vi "Execute.vi"(8 "error in (no error)":errorcluster, 11 "Node in":refnum<class "Set Double Float.lvclass">) -> (0 "error out":errorcluster, 1 "Status":T1, 3 "Node out":refnum<class "Set Double Float.lvclass">)   [LabVIEW 2021, in "BT.lvlib" / "Set Double Float.lvclass"]
uses:
  Set Double Float.lvclass
  C:/Users/Tim/Documents/GitHub/LV_Behaviour_Tree/BT Abstract Type/abs_Type Leaf/abs_Type Leaf.lvclass
  abs_Node/Status.ctl
  <vilib>/TSA/Abstract Data Classes/Abs_Types/Double Float/Abs_Double Float.lvclass
  C:/Program Files (x86)/National Instruments/LabVIEW 2021/vi.lib/TSA/Abstract Data Classes/Abs_Types/Type/Abs_Type.lvclass
  abs_Type Leaf/abs_Type Leaf.lvclass/abs_Type Leaf.ctl
  Set Double Float.lvclass/Set Double Float.ctl
  abs_Type Leaf/Properties/Read Value Class.vi
  Properties/Read Value.vi
  abs_Type Leaf/Properties/Write Value Class.vi
  <vilib>/TSA/Abstract Data Classes/Abs_Types/Type/Abs_Type.lvclass
  abs_Type Leaf/abs_Type Leaf.lvclass
  abs_Node/bt_Node.lvclass
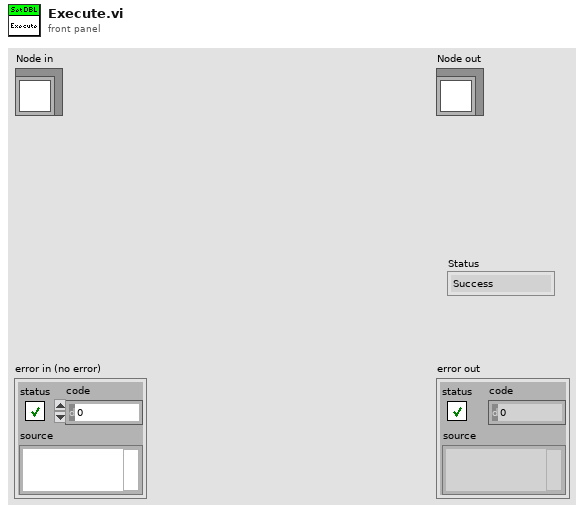
[diagram p1: front panel]
types:
  T1 = typedef "BT.lvlib/bt_Node.lvclass/Status.ctl" = enum16{"Success", "Failure", "Running"}
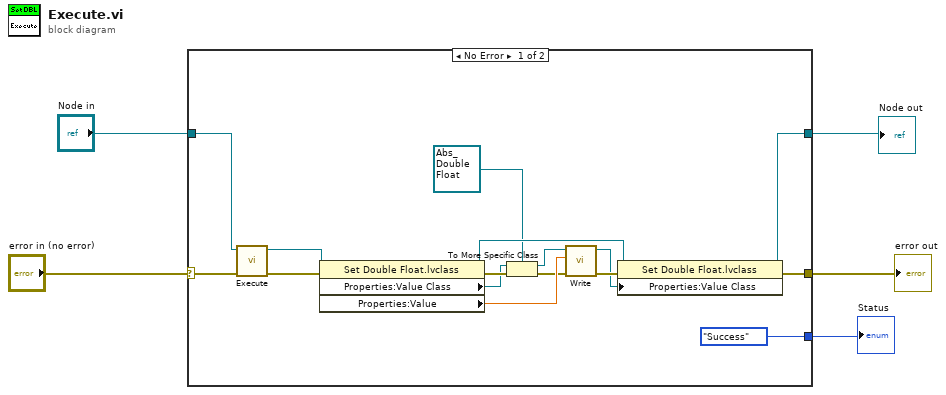
[diagram p0: block diagram]
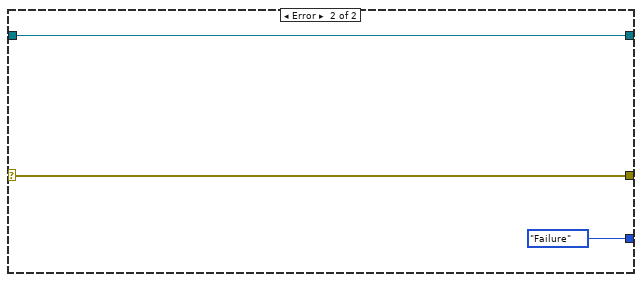
[diagram p2: hidden frame]
diagram:
  n1 = case shown="No Error" "error in (no error)" {
    selector: "error in (no error)" -> [w21 w23]
    tunnel: "Node in" -> [w20 w24]
    tunnel: [w16 w23] -> w4
    tunnel: [w15 w24] -> w2
    tunnel: [Status."Success" ("Status") Status."Failure" ("Status")] -> w3
    frame No Error {
      n2 = call-parent "Execute.vi"("error in (no error)"=w21, "Node in"=w20) -> ("error out"=w19:errorcluster, "Node out"=w18:refnum<class "Set Double Float.lvclass">)  [unwired: 7 in, 1 out]
      n3 = property class="Set Double Float.lvclass"(reference=w18, error in=w19) -> (reference out=w17:refnum<class "Set Double Float.lvclass">, error out=w10:errorcluster, "Properties:Value Class"=w8:refnum<class "Abs_Type.lvclass">, "Properties:Value"=w11:dbl)
      n4 = To More Specific Class(target class=refnum<class "Abs_Double Float.lvclass"> refnum ("Double Float.lvclass_340760 in"), reference=w8, error in=w10) -> (specific class reference=w6:refnum<class "Abs_Double Float.lvclass">, error out=w9:errorcluster)
      n5 = call-dynamic "Write.vi"("error in (no error)"=w9, "Value"=w11, "Double Float.lvclass in"=w6) -> ("error out"=w13:errorcluster, "Double Float.lvclass out"=w12:refnum<class "Abs_Double Float.lvclass">)  [unwired: 7 in]
      n6 = property class="Set Double Float.lvclass"(reference=w17, error in=w13, "Properties:Value Class"=w12) -> (reference out=w15:refnum<class "Set Double Float.lvclass">, error out=w16:errorcluster)
    }
    frame Error {
    }
  }
  "error out" <- w4
  "Node out" <- w2
  "Status" <- w3
